vi "CD Init_Prepare Async Data_BC Command Channels.vi"(8 "error in (no error)":errorcluster, 10 "Card Parameters (in)":T1, 11 "Channels In":T6[](array[typedef]) {"RTs"."Mode Codes"."Words Item Refs" format="%.0x"; "RTs"."Mode Codes"."Timestamp Channel Data Reference" format="%.0x"; "RTs"."subAddresses"."Words Item Refs" format="%.0x"; "RTs"."subAddresses"."Timestamp Channel Data Reference" format="%.0x"; "RTs"."Status Channel Data Reference" format="%.0x"; "RTs"."Command Channels Refs" format="%.0x"; "BC"."Acyclic Frames Trigger Channels Refs" format="%.0x"; "BC"."Command Channels Refs" format="%.0x"; "BC"."messages"."Timestamp Channel Data Reference" format="%.0x"; "BC"."messages"."Status Channel Data Refs" format="%.0x"; "BC"."messages"."Words Item Refs" format="%.0x"; "BC"."messages"."Words Block Data Refs"."Data Reference" format="%.0x"}) -> (0 "error out":errorcluster, 3 "Map (Bc Command Channels)":T3[](array[typedef]) {"BC Command Channel Ref" format="%.0x"})   [LabVIEW 2017, in "Ballard MIL-1553 Engine.lvlib"]
doc: "This VI creates a static association between NI-VS FIFO Channel Index and Physical Channel, Label Index, Parameter Index for Parameter Channel of a Tx Scheduled Label."
uses:
  Ballard MIL-1553 Engine.lvlib
  Shared/Controls and Global/RT Channel.ctl
  Shared/Controls and Global/RT BC.ctl
  <vilib>/NI Veristand/Custom Device API/Custom Device Item Ref.ctl
  Shared/Controls and Global/RT Message.ctl
  Shared/Controls and Global/RT messageType.ctl
  Shared/Controls and Global/RT CWD1.ctl
  Shared/Controls and Global/RT CWD2.ctl
  <vilib>/NI Veristand/Custom Device API/Data Reference.ctl
  <vilib>/NI Veristand/Custom Device API/Block Data Reference.ctl
  Shared/Controls and Global/RT Remote Terminal.ctl
  Shared/Controls and Global/RT Remote Terminal_rtMode.ctl
  Shared/Controls and Global/RT Remote Terminal_RT subAddress.ctl
  Shared/Controls and Global/RT Remote Terminal_RT direction.ctl
  Shared/Controls and Global/RT Remote Terminal_RT Mode Code.ctl
  Controls/RT Async_Map BC Command Channels.ctl
  Controls/RT Async_Map_Type.ctl
  Controls/Card Parameters.ctl
  Shared/Controls and Global/Initialization Method.ctl
  <instrlib>/BTI1553Lib/BTI1553LV.lvlib
  <vilib>/NI VeriStand/Custom Device API/Custom Device API.lvlib
  Shared/Ballard 1553 Shared.lvlib
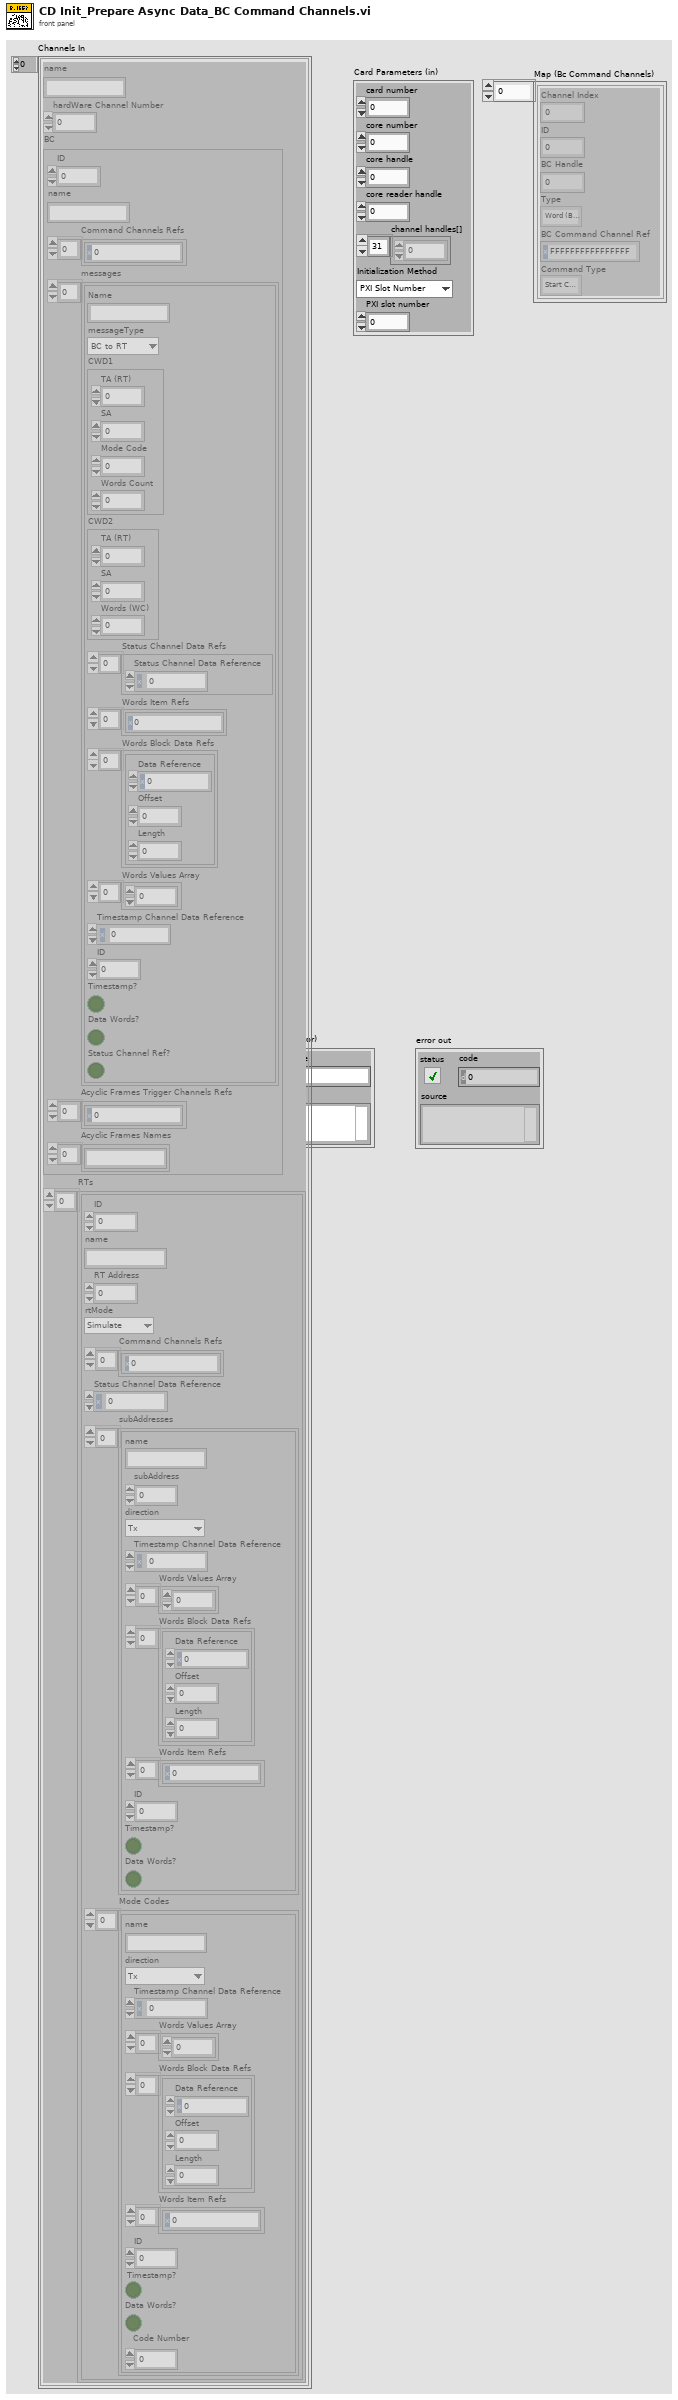
[diagram p1: front panel]
types:
  T1 = typedef "Ballard MIL-1553 Engine.lvlib/Card Parameters.ctl" = cluster{"card number":i32, "core number":i32, "core handle":u64, "core reader handle":u64, "channel handles[]":u64[], "Initialization Method":T2, "PXI slot number":i32}
  T2 = typedef "Ballard 1553 Shared.lvlib/Initialization Method.ctl" = enum16{"PXI Slot Number", "Card Number"}
  T3 = typedef "Ballard MIL-1553 Engine.lvlib/RT Async_Map BC Command Channels.ctl" = cluster{"Channel Index":i32, "ID":i32, "BC Handle":u64, "Type":T4, "BC Command Channel Ref":T5, "Command Type":enum16{"Start Command", "Stop Command"}}
  T4 = typedef "Ballard MIL-1553 Engine.lvlib/RT Async_Map_Type.ctl" = enum16{"Word (BC to RT)", "Word (MC (Rx))", "Acyclic Message Trigger", "Word (RT to ..)", "Word (RT to RT)", "Word (MC (Tx))", "RT Status", "BC Commands", "RT Commands"}
  T5 = typedef "Custom Device API.lvlib/Custom Device Item Ref.ctl" = u64
  T6 = typedef "Ballard 1553 Shared.lvlib/RT Channel.ctl" = cluster{"name":string, "hardWare Channel Number":u16, "BC":T7, "RTs":T14[]}
  T7 = typedef "Ballard 1553 Shared.lvlib/RT BC.ctl" = cluster{"ID":i32, "name":string, "Command Channels Refs":T5[], "messages":T8[], "Acyclic Frames Trigger Channels Refs":T5[], "Acyclic Frames Names":string[]}
  T8 = typedef "Ballard 1553 Shared.lvlib/RT Message.ctl" = cluster{"Name":string, "messageType":T9, "CWD1":T10, "CWD2":T11, "Status Channel Data Refs":T12[], "Words Item Refs":T5[], "Words Block Data Refs":T13[], "Words Values Array":u16[], "Timestamp Channel Data Reference":T12, "ID":i32, "Timestamp?":bool, "Data Words?":bool, "Status Channel Ref?":bool}
  T9 = typedef "Ballard 1553 Shared.lvlib/RT messageType.ctl" = enum16{"BC to RT", "RT to BC", "RT to RT", "MC (Rx)", "MC (Tx)"}
  T10 = typedef "Ballard 1553 Shared.lvlib/RT CWD1.ctl" = cluster{"TA (RT)":i8, "SA":i8, "Mode Code":i8, "Words Count":i8}
  T11 = typedef "Ballard 1553 Shared.lvlib/RT CWD2.ctl" = cluster{"TA (RT)":i8, "SA":i8, "Words (WC)":i8}
  T12 = typedef "Custom Device API.lvlib/Data Reference.ctl" = i32
  T13 = typedef "Custom Device API.lvlib/Block Data Reference.ctl" = cluster{"Data Reference":T12, "Offset":u64, "Length":u64}
  T14 = typedef "Ballard 1553 Shared.lvlib/RT Remote Terminal.ctl" = cluster{"ID":i32, "name":string, "RT Address":i32, "rtMode":T15, "Command Channels Refs":T5[], "Status Channel Data Reference":T12, "subAddresses":T16[], "Mode Codes":T18[]}
  T15 = typedef "Ballard 1553 Shared.lvlib/RT Remote Terminal_rtMode.ctl" = enum16{"Simulate", "Monitor", "Disable"}
  T16 = typedef "Ballard 1553 Shared.lvlib/RT Remote Terminal_RT subAddress.ctl" = cluster{"name":string, "subAddress":i8, "direction":T17, "Timestamp Channel Data Reference":T12, "Words Values Array":u16[], "Words Block Data Refs":T13[], "Words Item Refs":T5[], "ID":i32, "Timestamp?":bool, "Data Words?":bool}
  T17 = typedef "Ballard 1553 Shared.lvlib/RT Remote Terminal_RT direction.ctl" = enum16{"Tx", "Rx"}
  T18 = typedef "Ballard 1553 Shared.lvlib/RT Remote Terminal_RT Mode Code.ctl" = cluster{"name":string, "direction":T17, "Timestamp Channel Data Reference":T12, "Words Values Array":u16[], "Words Block Data Refs":T13[], "Words Item Refs":T5[], "ID":i32, "Timestamp?":bool, "Data Words?":bool, "Code Number":i32}
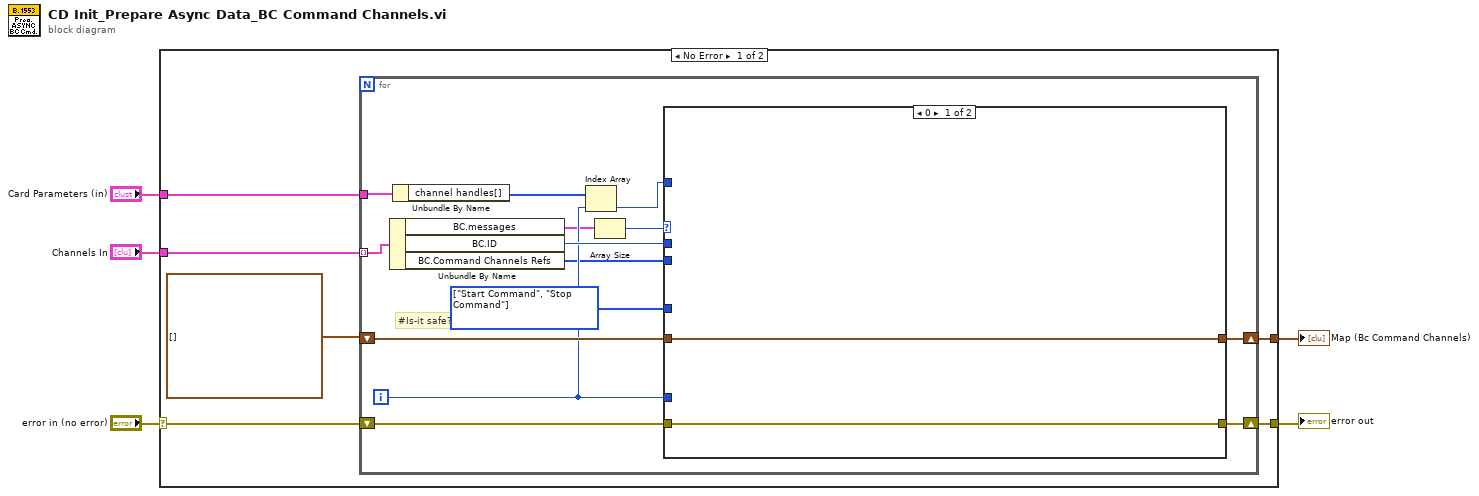
[diagram p0: block diagram]
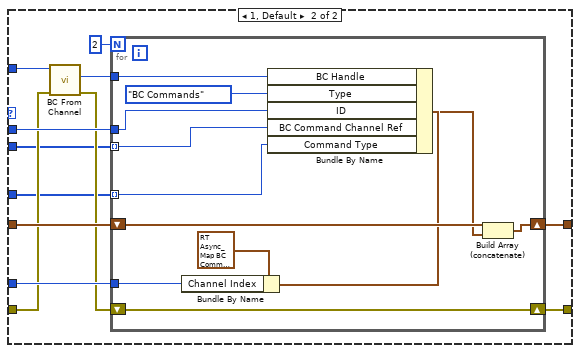
[diagram p2: hidden frame]
diagram:
  n1 = case shown="No Error" "error in (no error)" {
    selector: "error in (no error)" -> [w7 w52]
    tunnel: [w6 w52] -> w4
    tunnel: "Channels In" -> [w11 _]
    tunnel: [w9 _] -> w2
    tunnel: "Card Parameters (in)" -> [w8 _]
    frame No Error {
      n2 = for {
        tunnel: w11 -> [w24] mode=indexing
        shift-right: [w22] -> w9
        shift-left: T3[] [] -> [w23]
        tunnel: w8 -> [w21]
        shift-right: [w18] -> w6
        shift-left: w7 -> [w16]
        i -> [w19]
        w14 = enum16{"Start Command", "Stop Command"}[] [enum."Start Command", enum."Stop Command"] items=["Start Command", "Stop Command"]
        # "#Is-it safe?"
        n3 = Unbundle By Name(w24) -> ("BC.messages"=w13:T8[], "BC.ID"=w25:i32, "BC.Command Channels Refs"=w15:T5[])
        n4 = Unbundle By Name(w21) -> ("channel handles[]"=w20:u64[])
        n5 = Index Array(array=w20, index=w19) -> (element=w17:u64)
        n6 = Array Size(array=w13) -> (size(s)=w12:i32)
        n7 = case shown="0" w12 {
          tunnel: w25 -> [_ w39]
          tunnel: w23 -> [w27 w38]
          tunnel: [w27 w37] -> w22
          tunnel: w19 -> [_ w36]
          tunnel: [w26 w35] -> w18
          tunnel: w17 -> [_ w34]
          tunnel: w16 -> [w26 w33]
          tunnel: w15 -> [_ w30]
          tunnel: w14 -> [_ w28]
          frame 0 {
          }
          frame 1, Default {
            n8 = call <instrlib>:"BC From Channel.vi"("error in (no error)"=w33, "channel handle in"=w34) -> ("error out"=w32:errorcluster, "bus controller handle out"=w31:u64)  [unwired: 7 in, 1 out]
            n9 = for {
              N: 2 -> [_]
              tunnel: w39 -> [w43]
              shift-right: [w50] -> w37
              shift-left: w38 -> [w49]
              tunnel: w36 -> [w51]
              tunnel: w31 -> [w48]
              shift-right: [w42] -> w35
              shift-left: w32 -> [w42]
              tunnel: w30 -> [w40] mode=indexing
              tunnel: w28 -> [w41] mode=indexing
              n10 = Bundle By Name(cluster=T3 {"Channel Index"=0, "ID"=0, "BC Handle"=0, "Type"=enum."Word (BC to RT)", "BC Command Channel Ref"=18446744073709551615, "Command Type"=enum."Start Command"} ("Association"), "Channel Index"=w51) -> (w47:T3)
              n11 = Bundle By Name(cluster=w47, "BC Handle"=w48, "Type"=RT_Async_Map_Type."BC Commands", "ID"=w43, "BC Command Channel Ref"=w40, "Command Type"=w41) -> (w45:T3)
              n12 = Build Array (concatenate)(w49, w45) -> (w50:T3[])
            }
          }
        }
      }
    }
    frame Error {
    }
  }
  "error out" <- w4
  "Map (Bc Command Channels)" <- w2
